vi "Main.vi"(8 "error in (no error)":errorcluster, 9 "duty cycle [%]":dbl, 10 "freq [Hz]":dbl=50.0, 11 "PWM channel 2":tag="B/PWM0") -> (0 "error out":errorcluster)   [LabVIEW 2017]
uses:
  <vilib>/myRIO/Common/Instrument Driver Framework/myRIO v1.0/PWM/vis/myRIO v1.1 Open PWM.vi
  <vilib>/myRIO/Common/Instrument Driver Framework/myRIO v1.0/UART/vis/myRIO v1.0 Close UART.vi
  <vilib>/myRIO/Common/Instrument Driver Framework/Utilities/vis/Validate Channels.vi
  <vilib>/myRIO/Common/Instrument Driver Framework/myRIO v1.0/PWM/vis/myRIO v1.0 Reserve PWM.vi
  <vilib>/myRIO/Common/Instrument Driver Framework/myRIO v1.0/PWM/vis/myRIO v1.0 Build MUX Configuration PWM.vi
  <vilib>/myRIO/Common/Instrument Driver Framework/myRIO v1.0/Resource Manager/vis/myRIO v1.0 Reserve Channel List.vi
  <vilib>/myRIO/Common/Instrument Driver Framework/myRIO v1.0/Resource Manager/vis/myRIO v1.0 Create Configuration List.vi
  <vilib>/myRIO/Common/Instrument Driver Framework/myRIO v1.0/Resource Manager/vis/myRIO v1.0 Reserve Channel.vi
  <vilib>/myRIO/Common/Instrument Driver Framework/myRIO v1.0/Resource Manager/vis/myRIO v1.0 Unreserve Channel.vi
  <vilib>/myRIO/Common/Instrument Driver Framework/myRIO v1.0/Resource Manager/vis/myRIO v1.0 Build Mutex Name.vi
  <vilib>/Utility/VariantDataType/GetNumericInfo.vi
  <vilib>/Utility/error.llb/Error Cluster From Error Code.vi
  <vilib>/myRIO/Common/Instrument Driver Framework/myRIO v1.0/myRIO v1.1 Open.vi
  <vilib>/myRIO/Common/Instrument Driver Framework/Utilities/vis/IO Manager.vi
  <vilib>/myRIO/Common/Instrument Driver Framework/Utilities/vis/Configuration Manager.vi
  <vilib>/myRIO/Common/Instrument Driver Framework/myRIO v1.0/Resource Manager/vis/myRIO v1.0 Configure IO.vi
  <vilib>/myRIO/Common/Instrument Driver Framework/myRIO v1.0/myRIO v1.0 Close.vi
  <vilib>/myRIO/Common/Instrument Driver Framework/myRIO v1.0/PWM/vis/myRIO v1.0 Write PWM.vi
  <vilib>/myRIO/Common/Instrument Driver Framework/Utilities/vis/FPGA Ref Manager.vi
  <vilib>/myRIO/Common/Instrument Driver Framework/myRIO v1.0/myRIO v1.0 Reset FPGA.vi
  <vilib>/myRIO/Common/Instrument Driver Framework/myRIO v1.0/IRQ/vis/myRIO v1.0 IRQ Info FGV.vi
  <vilib>/myRIO/Common/Instrument Driver Framework/myRIO v1.0/IRQ/vis/myRIO v1.0 Timer IRQ Info FGV.vi
  <vilib>/myRIO/Common/Instrument Driver Framework/myRIO v1.0/IRQ/vis/myRIO v1.0 ISR Agent.vi
  <vilib>/myRIO/Instrument Drivers/Utilities/Utilities.lvlib
  <vilib>/myRIO/Instrument Drivers/Onboard IO/PWM/PWM.lvlib
panel:
  in  "[ESC] 2":bool
  # "Servo"
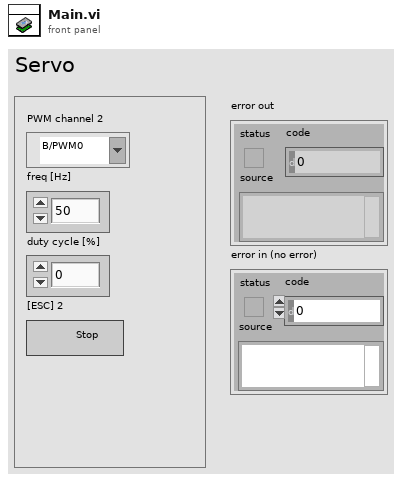
[diagram p1: front panel]
types:
  T1 = typedef "PWM.lvlib/PWM Reference.ctl" = cluster{"myRIO Reference":T2, "PWM Channels Enum":T6, "PWM Configuration":T7}
  T2 = typedef "myRIO Generic Hardware Reference.ctl" = cluster{"myRIO Model":T3, "myRIO Hardware Reference":T4}
  T3 = typedef "Hardware Version Enum.ctl" = enum16{"Unknown", "myRIO-1900", "myRIO-1950", "roboRIO", "NI ELVIS RIO CM"}
  T4 = typedef "myRIO v1.0 Reference.ctl" = cluster{"Generic FPGA Reference":T5, "Allow multiple opens":bool}
  T5 = typedef "Generic FPGA Reference.ctl" = refnum<k20>
  T6 = typedef "PWM Channels Enum.ctl" = enum16{"Not Connected", "C/PWM0", "C/PWM1", "A/PWM0", "A/PWM1", "A/PWM2", "B/PWM0", "B/PWM1", "B/PWM2", "PWM/PWM0", "PWM/PWM1", "PWM/PWM2", "PWM/PWM3", "PWM/PWM4", "PWM/PWM5", "PWM/PWM6", "PWM/PWM7", "PWM/PWM8", "PWM/PWM9"}
  T7 = typedef "PWM.lvlib/PWM Configuration.ctl" = cluster{"Frequency":dbl, "Duty Cycle":dbl}
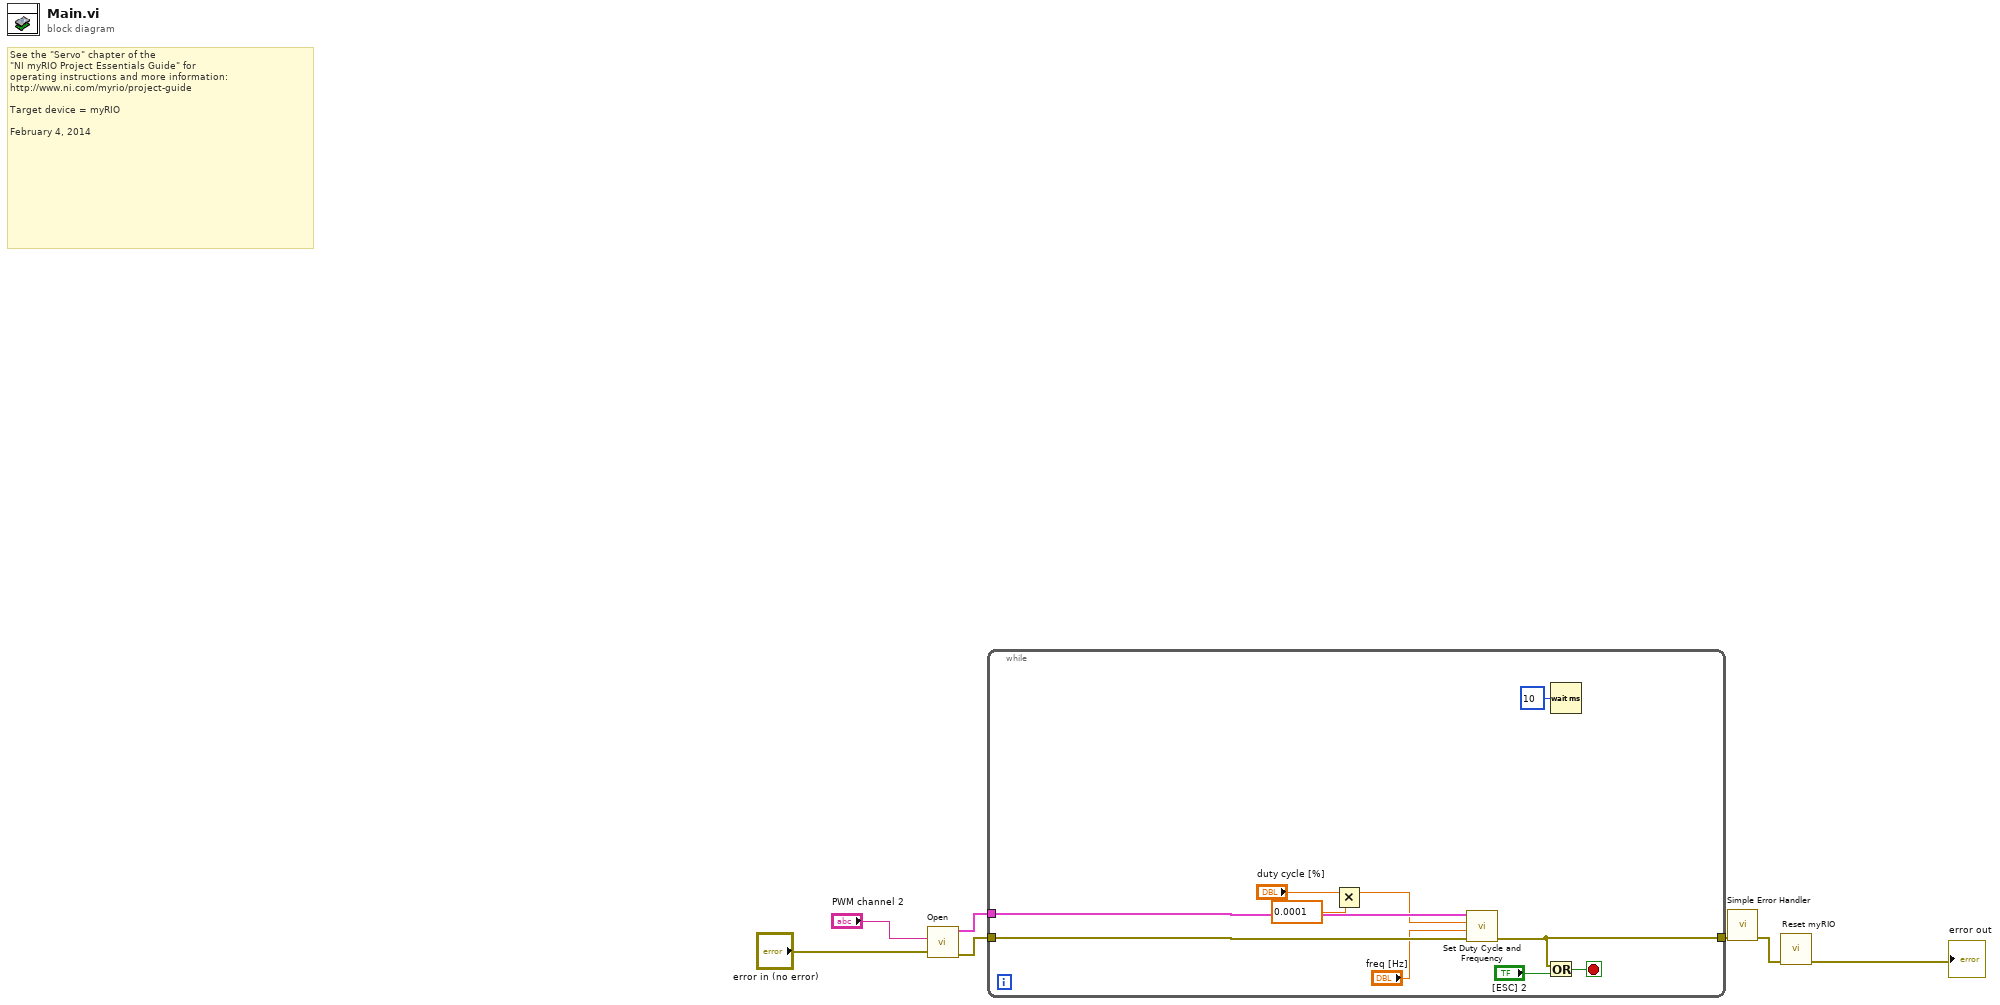
[diagram p0: block diagram]
diagram:
  # "See the \"Servo\" chapter of the\n\"NI myRIO Project Essentials Guide\" for\noperating instructions and more information: \nhttp://www.ni.com/myrio/project-guide\n\nTarget device = myRIO\n\nFebruary 4, 2014"
  n1 = call <vilib>:"Open.vi"("error in (no error)"="error in (no error)", "Channel Name"="PWM channel 2") -> ("error out"=w4:errorcluster, "PWM Ref Out"=w5:T1)  [unwired: 8 in]
  n2 = while {
    tunnel: w5 -> [w14]
    tunnel: w4 -> [w13]
    tunnel: [w12] -> w3
    stop <- w17 stop-if-true
    n3 = Multiply(x="duty cycle [%]", y=0.0001) -> (x*y=w9:dbl)
    n4 = call <vilib>:"Set Duty Cycle and Frequency.vi"("error in (no error)"=w13, "Frequency [Hz]"="freq [Hz]", "Duty Cycle"=w9, "PWM Ref In"=w14) -> ("error out"=w12:errorcluster)  [unwired: 5 in, 1 out]
    n5 = Or(x=w12, y="[ESC] 2") -> (x .or. y?=w17:bool)
    n6 = Wait (ms)(milliseconds to wait=u32 10) -> ()  [unwired: 1 out]
  }
  n7 = call <vilib>:"Simple Error Handler.vi"("error in (no error)"=w3) -> ("error out"=w7:errorcluster)  [unwired: 4 in, 4 out]
  n8 = call <vilib>:"Reset myRIO.vi"("error in (no error)"=w7) -> ("error out"=→"error out":errorcluster)  [unwired: 10 in]
